vi "NI VeriStand - Set Aliases.vi"(7 "Runtime Alias Folder Name":string, 8 "Error in":errorcluster, 9 "Alias Names":string[](array[string]), 10 "Referenced Channels":string[](array[string]), 11 "Runtime Configuration Ref in":refnum<k24>) -> (0 "Error out":errorcluster, 1 "Alias Names":string[](array[string]), 2 "Referenced Channels":string[](array[string]), 3 "Runtime Configuration Ref out":refnum<k24>, 5 "Success":bool)   [LabVIEW 2026, in "NI_VS RuntimeConfigurationFile ScriptingAPI.lvlib"]
uses:
  NI_VS RuntimeConfigurationFile ScriptingAPI.lvlib
  NationalInstruments.VeriStand.SystemDefinitionAPI
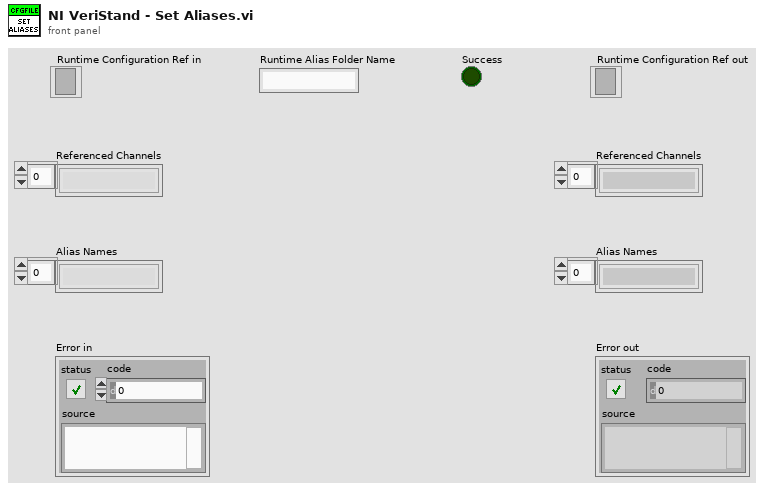
[diagram p1: front panel]
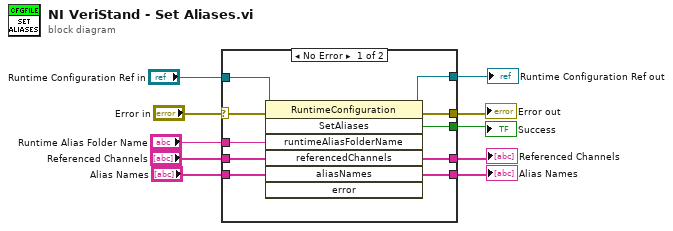
[diagram p0: block diagram]
diagram:
  n1 = case shown="No Error" "Error in" {
    selector: "Error in" -> [w19 w21]
    tunnel: "Runtime Configuration Ref in" -> [w18 _]
    tunnel: "Runtime Alias Folder Name" -> [w17 _]
    tunnel: "Referenced Channels" -> [w16 _]
    tunnel: "Alias Names" -> [w15 _]
    tunnel: [w14 _] -> w4
    tunnel: [w20 w21] -> w10
    tunnel: [w13 _] -> w3
    tunnel: [w12 _] -> w2
    tunnel: [w11 _] -> w1
    frame No Error {
      n2 = invoke class="RuntimeConfiguration" method="SetAliases"(reference=w18, error in=w19, "runtimeAliasFolderName"=w17, "referencedChannels"=w16, "aliasNames"=w15) -> (reference out=w14:refnum<k24>, error out=w20:errorcluster, "SetAliases"=w13:bool, "referencedChannels"=w12:string[], "aliasNames"=w11:string[])  [unwired: 2 in, 2 out]
    }
    frame Error {
    }
  }
  "Runtime Configuration Ref out" <- w4
  "Error out" <- w10
  "Success" <- w3
  "Referenced Channels" <- w2
  "Alias Names" <- w1
